vi "CTU.vi"(4 "R":bool, 6 "DI":u32, 7 "IN":bool) -> (1 "DO":u32, 2 "EU":bool)   [LabVIEW 2019, in "Counter.lvlib"]
uses:
  Counter.lvlib
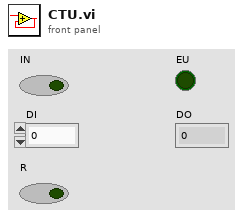
[diagram p1: front panel]
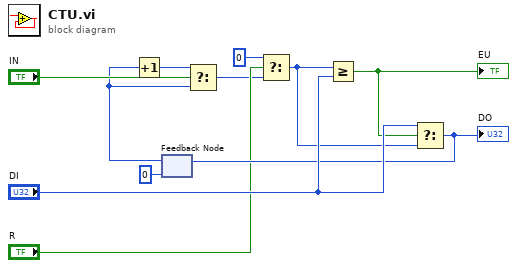
[diagram p0: block diagram]
diagram:
  n1 = feedback #1(u32 0) -> (w2:u32)
  n2 = Increment(x=w2) -> (x+1=w3:u32)
  n3 = Select(t=w3, s="IN", f=w2) -> (s? t:f=w1:u32)
  n4 = Select(t=u32 0, s="R", f=w1) -> (s? t:f=w5:u32)
  n5 = Greater Or Equal?(x=w5, y="DI") -> (x >= y?=w9:bool)
  "EU" <- w9
  n6 = Select(t="DI", s=w9, f=w5) -> (s? t:f=w8:u32)
  "DO" <- w8
  n7 = feedback-in #1(w8) -> ()
